vi "SVD.vi"(11 "data (scaled)":dbl[][](array[numeric])) -> (2 "v":dbl[][](array[numeric]), 3 "d":dbl[](array[numeric]))   [LabVIEW 2014]
uses:
  <vilib>/Analysis/7linalg.llb/Eigenvalue and Vectors Output Option.ctl
  <vilib>/Analysis/baseanly.llb/Real A x B.vi
  <vilib>/Analysis/7linalg.llb/Real Eigenvalues and Vectors.vi
  <vilib>/Analysis/Matrix/Numeric/Conversions/Matrix To Array - CM.vi
  <vilib>/Analysis/7linalg.llb/Real SVD Decomposition.vi
  <vilib>/Analysis/NI_AALPro.lvlib
  <vilib>/Analysis/NI_AALBase.lvlib
  <vilib>/Analysis/Matrix/NI_Matrix.lvlib
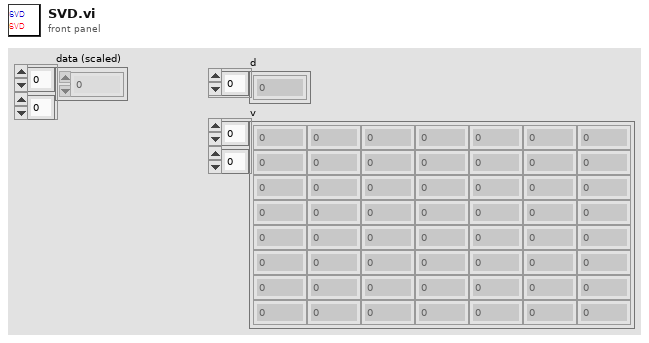
[diagram p1: front panel]
types:
  T1 = typedef "NI_AALPro.lvlib/Eigenvalue and Vectors Output Option.ctl" = i32
  T2 = typedef "NI_Matrix.lvlib/RealMatrix.ctl" = dbl[][]
  T3 = typedef "NI_Matrix.lvlib/ComplexMatrix.ctl" = cdb[][]
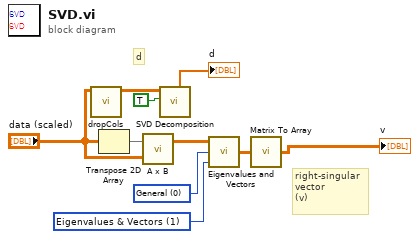
[diagram p0: block diagram]
diagram:
  w9 = T1 1 items=["Eigenvalues", "Eigenvalues & Vectors"] ("output option")
  w8 = 0 items=["General", "Symmetric"] ("matrix type")
  # "right-singular\nvector\n(v)"
  # "d"
  n1 = call "dropCols.vi"("data"="data (scaled)") -> ("data (columns dropped)"=w6:dbl[][])  [unwired: 10 in]
  n2 = Transpose 2D Array(2D array="data (scaled)") -> (transposed array=w2:dbl[][])
  n3 = call-poly <vilib>:"A x B.vi"("B"="data (scaled)", "A"=w2) -> ("A x B"=w7:T2)  [unwired: 1 out]
  n4 = call-poly <vilib>:"SVD Decomposition.vi"("singular values only?"=TRUE, "A"=w6) -> ("Vector S"=→"d":dbl[])  [unwired: 5 in, 4 out]
  n5 = call-poly <vilib>:"Eigenvalues and Vectors.vi"("output option"=w9, "matrix type"=w8, "Input Matrix"=w7) -> ("Eigenvectors"=w10:T3)  [unwired: 2 out]
  n6 = call-poly <vilib>:"Matrix To Array.vi"("Complex Matrix"=w10) -> ("Complex 2D Array"=→"v":cdb[][])
